vi "Get Initialize Edit Project.vi"(8 "error in (no error)":errorcluster, 11 "Abstract Initialize Edit Project Msg in":refnum<class "Abstract Initialize Edit Project Msg.lvclass">) -> (0 "error out":errorcluster, 2 "Initialize Edit Project":bool, 3 "Abstract Initialize Edit Project Msg out":refnum<class "Abstract Initialize Edit Project Msg.lvclass">)   [LabVIEW 2013, in "Edit Project Model.lvlib" / "Abstract Initialize Edit Project Msg.lvclass"]
uses:
  Abstract Initialize Edit Project Msg.lvclass
  Abstract Initialize Edit Project Msg.lvclass/Abstract Initialize Edit Project Msg.ctl
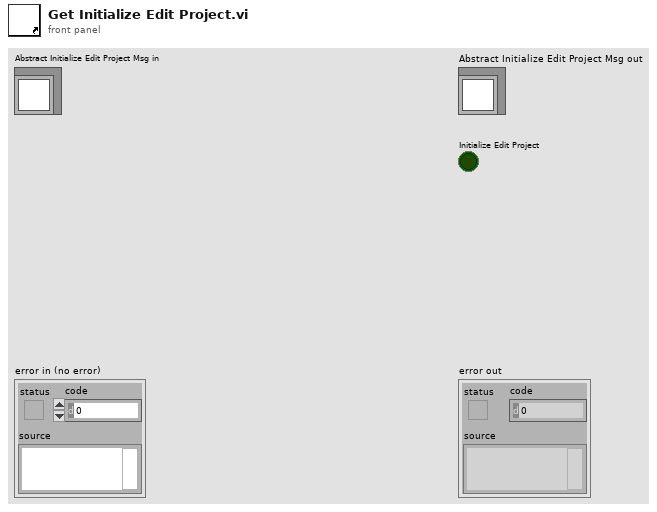
[diagram p1: front panel]
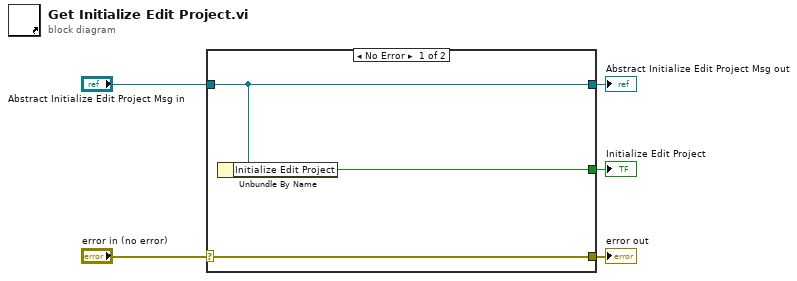
[diagram p0: block diagram]
diagram:
  n1 = case shown="No Error" "error in (no error)" {
    selector: "error in (no error)" -> [w8 w9]
    tunnel: [w8 w9] -> w4
    tunnel: [w7 w10] -> w2
    tunnel: "Abstract Initialize Edit Project Msg in" -> [w7 w10]
    tunnel: [w6 _] -> w1
    frame No Error {
      n2 = Unbundle By Name(w7) -> ("Initialize Edit Project"=w6:bool)
    }
    frame Error {
    }
  }
  "error out" <- w4
  "Abstract Initialize Edit Project Msg out" <- w2
  "Initialize Edit Project" <- w1
